vi "WSVCAP SHL Host LL SPI_RFFE Build Socket Mask.vi"(0 "DUT Mask":bool[](array[boolean])) -> (4 "Socket Mask [U64]":u64 format="%08x")   [LabVIEW 2012]
panel:
  # "DUT 01"
  # "DUT 02"
  # "DUT 03"
  # "DUT 04"
  # "DUT 05"
  # "DUT 06"
  # "DUT 07"
  # "DUT 08"
  # "DUT 09"
  # "DUT 10"
  # "DUT 11"
  # "DUT 12"
  # "DUT 13"
  # "DUT 14"
  # "DUT 15"
  # "DUT 16"
  # "DUT 17"
  # "DUT 18"
  # "DUT 19"
  # "DUT 20"
  # "DUT 21"
  # "DUT 22"
  # "DUT 23"
  # "DUT 24"
  # "DUT 25"
  # "DUT 26"
  # "DUT 27"
  # "DUT 28"
  # "DUT 29"
  # "DUT 30"
  # "DUT 31"
  # "DUT 32"
  # "DUT 33"
  # "DUT 34"
  # "DUT 35"
  # "DUT 36"
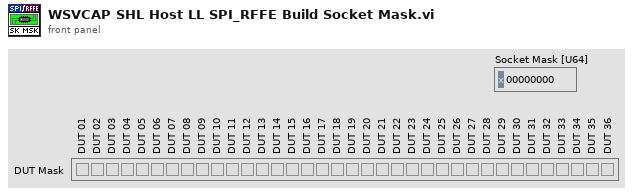
[diagram p1: front panel]
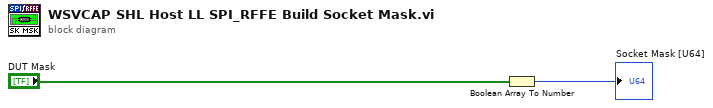
[diagram p0: block diagram]
diagram:
  n1 = Boolean Array To Number(Boolean array="DUT Mask") -> (number=→"Socket Mask [U64]":u64)
